vi "rad_Deploy Images in Parallel.vi"(4 "Deploy":string[](array[string]), 6 "restart after imaging (T)":bool=TRUE, 7 "Deployment Notifiers":T3[](array[typedef]), 8 "error in (no error)":errorcluster, 9 "apply primary NIC from image (F)":bool, 10 "image file path in":path, 11 "Target addresses in":T1[](array[typedef]) {"Primary NIC"."IP Address Request Mode" items=["Static"=1, "DHCP/Link-Local"=2, "Link-Local Only"=4, "DHCP Only"=8]}) -> (0 "Errors Out":errorcluster[](array[cluster]), 2 "image file path out":path, 3 "Target addresses out":T1[](array[typedef]) {"Primary NIC"."IP Address Request Mode" items=["Static"=1, "DHCP/Link-Local"=2, "Link-Local Only"=4, "DHCP Only"=8]})   [LabVIEW 2020]
uses:
  TypeDefs/rad_Deployment Notifiers.ctl
  TypeDefs/rad_Deployment Status Data Type.ctl
  TypeDefs/rad_Deployment Progress Data Type.ctl
  Targets/TypeDefs/rad_Target Information.ctl
  Targets/TypeDefs/rad_Target Network Settings.ctl
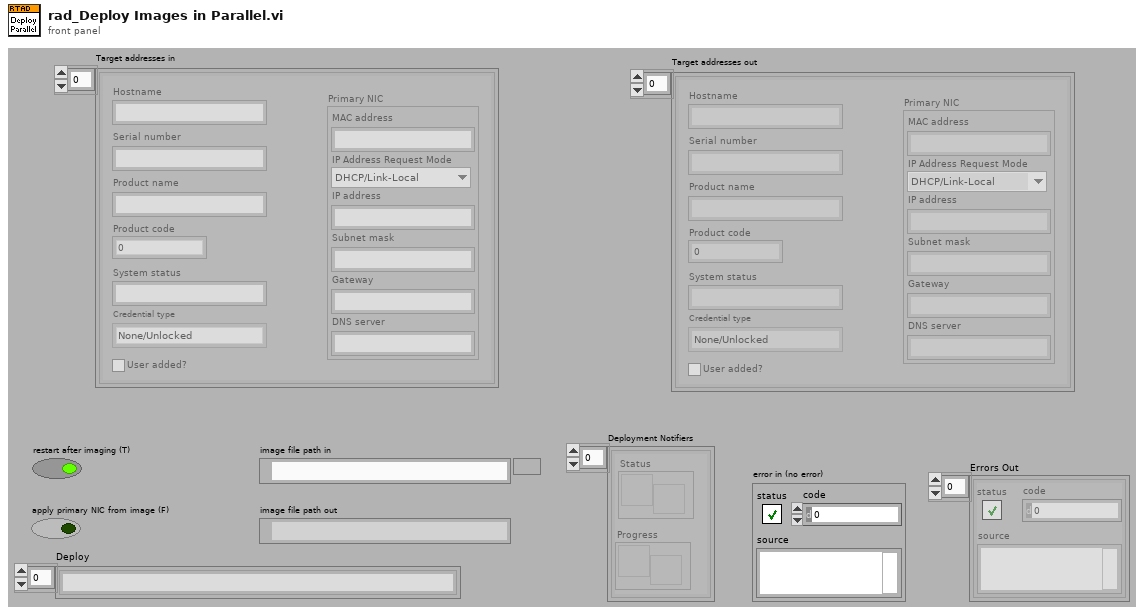
[diagram p1: front panel]
types:
  T1 = typedef "rad_Target Information.ctl" = cluster{"Hostname":string, "Serial number":string, "Product name":string, "Product code":i32, "System status":string, "Credential type":enum16{"None/Unlocked", "FTP Password", "NIAuth Credentials"}, "User added?":bool, "Primary NIC":T2}
  T2 = typedef "rad_Target Network Settings.ctl" = cluster{"MAC address":string, "IP Address Request Mode":i32, "IP address":string, "Subnet mask":string, "Gateway":string, "DNS server":string}
  T3 = typedef "rad_Deployment Notifiers.ctl" = cluster{"Status":refnum<notifier>, "Progress":refnum<notifier>}
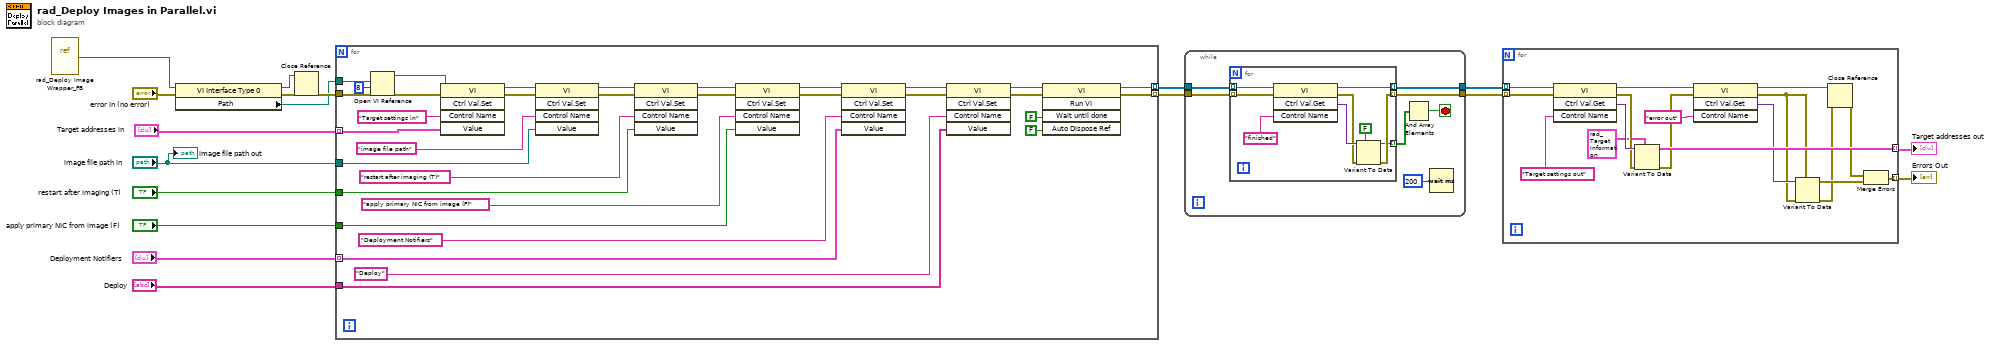
[diagram p0: block diagram]
diagram:
  n1 = vi-ref "rad_Deploy Image Wrapper_FB.vi"() -> (w1:refnum<vi>)
  n2 = property class="VI Interface Type 0"(reference=w1, error in="error in (no error)") -> (reference out=w18:refnum<vi>, error out=w17:errorcluster, "Path"=w15:path)
  n3 = Close Reference(reference=w18, error in (no error)=w17) -> (error out=w16:errorcluster)
  n4 = for {
    tunnel: w16 -> [w51]
    tunnel: w15 -> [w50]
    tunnel: "Target addresses in" -> [w46] mode=indexing
    tunnel: "image file path in" -> [w42]
    tunnel: "restart after imaging (T)" -> [w38]
    tunnel: [w35] -> w12 mode=indexing
    tunnel: [w34] -> w11 mode=indexing
    tunnel: "apply primary NIC from image (F)" -> [w29]
    tunnel: "Deployment Notifiers" -> [w26] mode=indexing
    tunnel: "Deploy" -> [w22]
    n5 = Open VI Reference(vi path=w50, options=8, error in (no error)=w51) -> (vi reference=w49:refnum<vi>, error out=w48:errorcluster)  [unwired: 3 in]
    n6 = invoke class="VI" method="Ctrl Val.Set"(reference=w49, error in=w48, "Control Name"="Target settings in", "Value"=w46) -> (reference out=w45:refnum<vi>, error out=w44:errorcluster)  [unwired: 1 in, 3 out]
    n7 = invoke class="VI" method="Ctrl Val.Set"(reference=w45, error in=w44, "Control Name"="image file path", "Value"=w42) -> (reference out=w41:refnum<vi>, error out=w40:errorcluster)  [unwired: 1 in, 3 out]
    n8 = invoke class="VI" method="Ctrl Val.Set"(reference=w41, error in=w40, "Control Name"="restart after imaging (T)", "Value"=w38) -> (reference out=w32:refnum<vi>, error out=w31:errorcluster)  [unwired: 1 in, 3 out]
    n9 = invoke class="VI" method="Ctrl Val.Set"(reference=w32, error in=w31, "Control Name"="apply primary NIC from image (F)", "Value"=w29) -> (reference out=w28:refnum<vi>, error out=w27:errorcluster)  [unwired: 1 in, 3 out]
    n10 = invoke class="VI" method="Ctrl Val.Set"(reference=w28, error in=w27, "Control Name"="Deployment Notifiers", "Value"=w26) -> (reference out=w20:refnum<vi>, error out=w21:errorcluster)  [unwired: 1 in, 3 out]
    n11 = invoke class="VI" method="Ctrl Val.Set"(reference=w20, error in=w21, "Control Name"="Deploy", "Value"=w22) -> (reference out=w25:refnum<vi>, error out=w24:errorcluster)  [unwired: 1 in, 3 out]
    n12 = invoke class="VI" method="Run VI"(reference=w25, error in=w24, "Wait until done"=FALSE ("Wait Until Done"), "Auto Dispose Ref"=FALSE ("Auto Dispose Reference")) -> (reference out=w35:refnum<vi>, error out=w34:errorcluster)  [unwired: 1 in, 3 out]
  }
  n13 = while {
    tunnel: w12 -> [w56]
    tunnel: w11 -> [w55]
    tunnel: [w53] -> w9
    tunnel: [w54] -> w10
    stop <- w57 stop-if-true
    n14 = for {
      tunnel: w56 -> [w67] mode=indexing
      tunnel: w55 -> [w66] mode=indexing
      tunnel: [w64] -> w54 mode=indexing
      tunnel: [w60] -> w53 mode=indexing
      tunnel: [w59] -> w52 mode=indexing
      n15 = invoke class="VI" method="Ctrl Val.Get"(reference=w67, error in=w66, "Control Name"="finished") -> (reference out=w64:refnum<vi>, error out=w61:errorcluster, "Get Control Value Variant"=w62:variant)  [unwired: 1 in, 1 out]
      n16 = Variant To Data(error in=w61, type=FALSE, Variant=w62) -> (data=w59:bool, error out=w60:errorcluster)
    }
    n17 = And Array Elements(Boolean array=w52) -> (logical AND=w57:bool)
    n18 = Wait (ms)(milliseconds to wait=u32 200) -> ()  [unwired: 1 out]
  }
  n19 = for {
    tunnel: w10 -> [w84] mode=indexing
    tunnel: w9 -> [w83] mode=indexing
    tunnel: [w80] -> w2 mode=indexing
    tunnel: [w72] -> w8 mode=indexing
    n20 = invoke class="VI" method="Ctrl Val.Get"(reference=w84, error in=w83, "Control Name"="Target settings out") -> (reference out=w79:refnum<vi>, error out=w78:errorcluster, "Get Control Value Variant"=w81:variant)  [unwired: 1 in, 1 out]
    n21 = Variant To Data(error in=w78, type=T1 {"Hostname"="", "Serial number"="", "Product name"="", "Product code"=0, "System status"="", "Credential type"=enum."None/Unlocked", "User added?"=FALSE, "Primary NIC"={"MAC address"="", "IP Address Request Mode"=0, "IP address"="", "Subnet mask"="", "Gateway"="", "DNS server"=""}} ("Target settings"), Variant=w81) -> (data=w80:T1, error out=w77:errorcluster)
    n22 = invoke class="VI" method="Ctrl Val.Get"(reference=w79, error in=w77, "Control Name"="error out") -> (reference out=w71:refnum<vi>, error out=w74:errorcluster, "Get Control Value Variant"=w75:variant)  [unwired: 1 in, 1 out]
    n23 = Variant To Data(error in=w74, type=w74, Variant=w75) -> (data=w73:errorcluster, error out=w70:errorcluster)
    n24 = Close Reference(reference=w71, error in (no error)=w70) -> (error out=w69:errorcluster)
    n25 = Merge Errors(w69, w73) -> (w72:errorcluster)
  }
  "Errors Out" <- w8
  "Target addresses out" <- w2
  "image file path out" <- "image file path in"
